vi "Set Control Caption Size and Pos Offset.vi"(9 "Caption.Font:Size":u32=14, 10 "Left Offset":i32=-10, 11 "Control in":refnum<vi>) -> ()   [LabVIEW 2019, in "Panther Dashboard.lvlib"]
uses:
  Panther Dashboard.lvlib
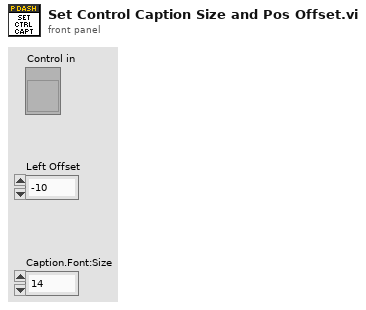
[diagram p1: front panel]
types:
  T1 = typedef "LVPositionTypeDef.ctl" = cluster{"Left":i32, "Top":i32}
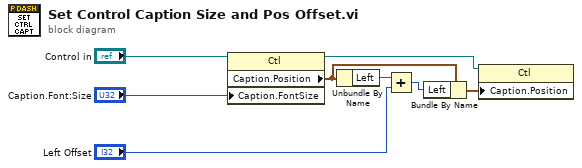
[diagram p0: block diagram]
diagram:
  n1 = property class="Ctl"(reference="Control in", "Caption.FontSize"="Caption.Font:Size") -> (reference out=w2:refnum<vi>, "Caption.Position"=w4:T1)  [unwired: 1 in, 1 out]
  n2 = Unbundle By Name(w4) -> ("Left"=w5:i32)
  n3 = Add(x=w5, y="Left Offset") -> (x+y=w6:i32)
  n4 = Bundle By Name(cluster=w4, "Left"=w6) -> (w3:T1)
  n5 = property class="Ctl"(reference=w2, "Caption.Position"=w3) -> ()  [unwired: 1 in, 2 out]
